vi "_Test_Data_In.vi"(10 "RC":i32, 11 "MsgID":i32 format="%x") -> (3 "Data_in":u8[](array[numeric]) format="%x")   [LabVIEW 2023, in "LP_CRC.lvlib"]
uses:
  LP_CRC.lvlib
panel:
  out "unsigned 8bit integer":u8 format="%x"
  out "element":u32 format="%x"
  out "value":u32[](array[numeric]) format="%x"
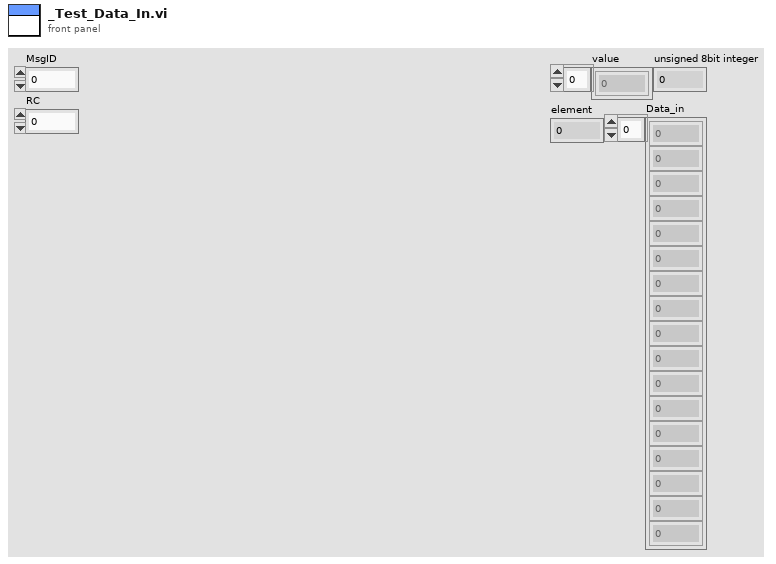
[diagram p1: front panel]
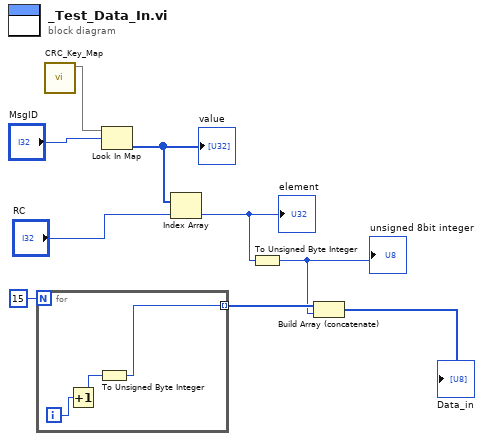
[diagram p0: block diagram]
diagram:
  n1 = for {
    N: 15 -> [_]
    tunnel: [w10] -> w4 mode=indexing
    i -> [w12]
    n2 = Increment(x=w12) -> (x+1=w11:i32)
    n3 = To Unsigned Byte Integer(number=w11) -> (unsigned 8bit integer=w10:u8)
  }
  n4 = call "CRC_Key_Map.vi"() -> ("Map"=w9:map{i32, u8[]})  [unwired: 11 in]
  n5 = Look In Map(map=w9, key="MsgID") -> (value=w7:u8[])  [unwired: 1 in, 1 out]
  "value" <- w7
  n6 = Index Array(array=w7, index="RC") -> (element=w3:u8)
  "element" <- w3
  n7 = To Unsigned Byte Integer(number=w3) -> (unsigned 8bit integer=w2:u8)
  "unsigned 8bit integer" <- w2
  n8 = Build Array (concatenate)(w4, w2) -> (→"Data_in":u8[])
